vi "Camera Intrinsics K.vi"(10 "Internal Parameters":T1) -> (1 "Camera intrinsic matrix (K^-1)":dbl[][](array[numeric])=[[-3.25, -3.25, 0.0], [3.25, -3.25, 0.0], [3.25, 3.25, 0.0], [-3.25, 3.25, 0.0]], 2 "Camera intrinsic matrix (K)":dbl[][](array[numeric])=[[-3.25, -3.25, 0.0], [3.25, -3.25, 0.0], [3.25, 3.25, 0.0], [-3.25, 3.25, 0.0]])   [LabVIEW 2025]
uses:
  <vilib>/vision/Calibration.llb/Internal Parameters.ctl
panel:
  out "fy":dbl
  out "fx":dbl
  out "cx width":dbl
  out "cy height":dbl
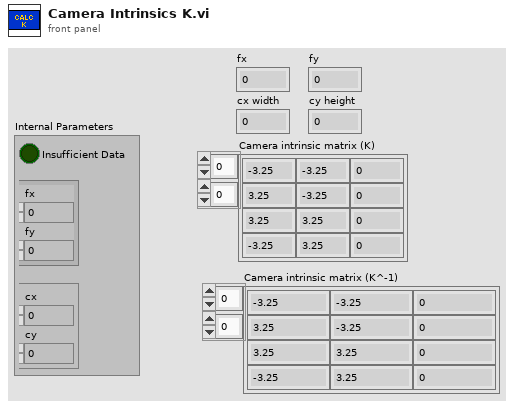
[diagram p1: front panel]
types:
  T1 = typedef "Internal Parameters.ctl" = cluster{"Insufficient Data":bool, "Focal Length (pixel)":cluster{"fx":sgl, "fy":sgl}, "Optical Center (pixel)":cluster{"cx":sgl, "cy":sgl}}
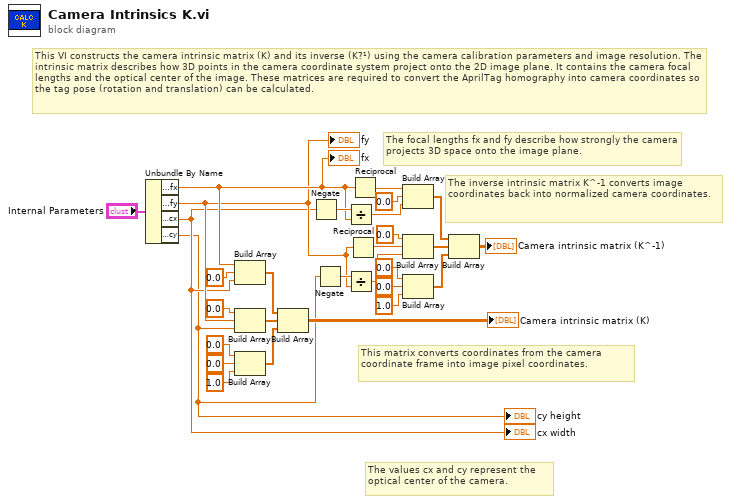
[diagram p0: block diagram]
diagram:
  # "The inverse intrinsic matrix K^-1 converts image coordinates back into normalized camera coordinates."
  # "This matrix converts coordinates from the camera coordinate frame into image pixel coordinates."
  # "The values cx and cy represent the optical center of the camera."
  # "The focal lengths fx and fy describe how strongly the camera projects 3D space onto the image plane."
  # "This VI constructs the camera intrinsic matrix (K) and its inverse (K?¹) using the camera calibration parameters and image resolution. The intrinsic matrix describes how 3D points in the camera coordinate system project onto the 2D image plane. It contains the camera focal lengths and the optical center of the image. These matrices are required to convert the AprilTag homography into camera coordinates so the tag pose (rotation and translation) can be calculated."
  n1 = Unbundle By Name("Internal Parameters") -> ("Focal Length (pixel).fx"=w4:sgl, "Focal Length (pixel).fy"=w3:sgl, "Optical Center (pixel).cx"=w2:sgl, "Optical Center (pixel).cy"=w1:sgl)
  "cy height" <- w1
  "cx width" <- w2
  "fx" <- w4
  "fy" <- w3
  n2 = Build Array(w4, 0.0 ("element"), w2) -> (w26:dbl[])
  n3 = Build Array(0.0 ("element"), w3, w1) -> (w27:dbl[])
  n4 = Build Array(0.0 ("element"), 0.0 ("element"), 1.0 ("element")) -> (w28:dbl[])
  n5 = Build Array(w26, w27, w28) -> (→"Camera intrinsic matrix (K)":dbl[][])
  n6 = Negate(x=w2) -> (-x=w12:sgl)
  n7 = Negate(x=w1) -> (-x=w10:sgl)
  n8 = Divide(x=w12, y=w4) -> (x/y=w13:sgl)
  n9 = Divide(x=w10, y=w3) -> (x/y=w9:sgl)
  n10 = Reciprocal(x=w3) -> (1/x=w6:sgl)
  n11 = Reciprocal(x=w4) -> (1/x=w7:sgl)
  n12 = Build Array(w7, 0.0 ("element"), w13) -> (w14:dbl[])
  n13 = Build Array(0.0 ("element"), w6, w9) -> (w15:dbl[])
  n14 = Build Array(0.0 ("element"), 0.0 ("element"), 1.0 ("element")) -> (w16:dbl[])
  n15 = Build Array(w14, w15, w16) -> (→"Camera intrinsic matrix (K^-1)":dbl[][])
